vi "LittleEndian_To_BigEndian.vi"(1 "Little Endian":u8[](array[numeric])) -> (0 "Big Endian":u8[](array[numeric]))   [LabVIEW 2015, in "navX Library v3.lvlib" / "navX Registry Cache.lvclass"]
uses:
  navX Registry Cache.lvclass
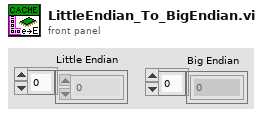
[diagram p1: front panel]
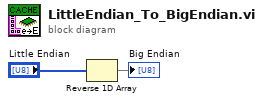
[diagram p0: block diagram]
diagram:
  n1 = Reverse 1D Array(array="Little Endian") -> (reversed array=→"Big Endian":u8[])
